vi "Initialize Instrument.vi"(8 "error in (no error)":errorcluster, 10 "Reset":bool, 11 "Agilent E4980 in":refnum<class "Agilent E4980.lvclass">) -> (0 "error out":errorcluster, 3 "Agilent E4980 out":refnum<class "Agilent E4980.lvclass">)   [LabVIEW 2020, in "Agilent E4980.lvclass"]
uses:
  Agilent E4980.lvclass
  C:/Sandbox/RF Bench/Source Code/WiSpry Test Framework/Instruments/Instrument.lvclass
  Instrument.lvclass/Instrument.ctl
  Instrument.lvclass
  <instrlib>/Agilent E4980/Agilent E4980.lvlib
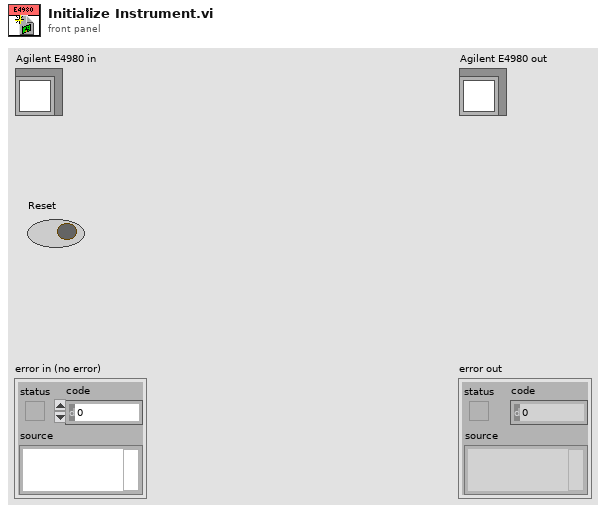
[diagram p1: front panel]
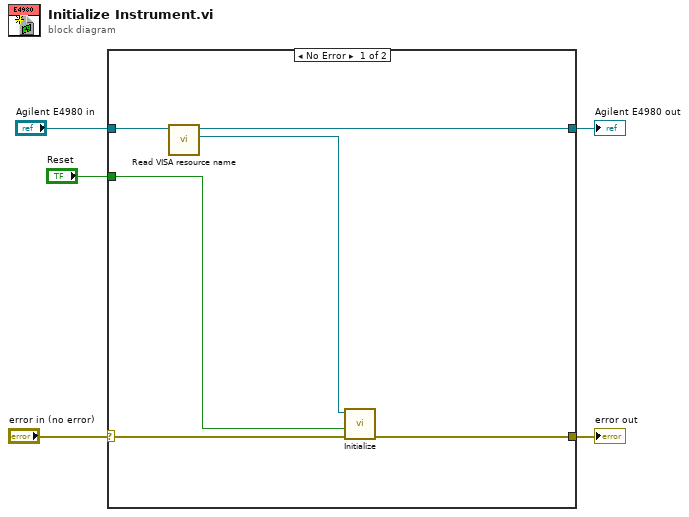
[diagram p0: block diagram]
diagram:
  n1 = case shown="No Error" "error in (no error)" {
    selector: "error in (no error)" -> [w9 w13]
    tunnel: [w6 w13] -> w2
    tunnel: [w10 w12] -> w1
    tunnel: "Agilent E4980 in" -> [w11 w12]
    tunnel: "Reset" -> [w8 _]
    frame No Error {
      n2 = call "Read VISA resource name.vi"("Instrument in"=w11) -> ("VISA resource name"=w7:refnum<visa-resource-name>, "Instrument out"=w10:refnum<class "Agilent E4980.lvclass">)  [unwired: 9 in]
      n3 = call <instrlib>:"Initialize.vi"("error in (no error)"=w9, "Reset (True)"=w8, "VISA resource name"=w7) -> ("error out"=w6:errorcluster)  [unwired: 7 in, 1 out]
    }
    frame Error {
    }
  }
  "error out" <- w2
  "Agilent E4980 out" <- w1
